vi "Main.vi"(5 "Deliminated Char":string=".", 6 "IGN Folder names":string[](array[string])=["StaARx#[PLC]StaATesterRxSignals", "StaATx#[PLC]StaATesterTxSignals"], 7 "IGN FGVname":string="OPC Ref", 8 "error in":errorcluster, 9 "Sequence Context In":refnum<k7>, 10 "Event Sources":T3, 11 "Ignition In":refnum<class "Ignition.lvclass">) -> (0 "error out":errorcluster, 2 "Station":string="asdfasdf", 3 "Ignition Out":refnum<class "Ignition.lvclass">)   [LabVIEW 2021, in "OPC UA.lvlib" / "Ignition.lvclass"]
uses:
  Ignition.lvclass
  Ignition.lvclass/Ignition.ctl
  OPC UA/OPC UA.lvclass
  Controls/Tester Rx.ctl
  Controls/Tester Tx.ctl
  <vilib>/addons/TestStand/_TSUtility.llb/TestStand - Get Property Value (Number {Signed 32-bit Integer}).vi
panel:
  out "Connect?":bool
  out "Tester Rx":T1
  in  "Tester Tx":T2
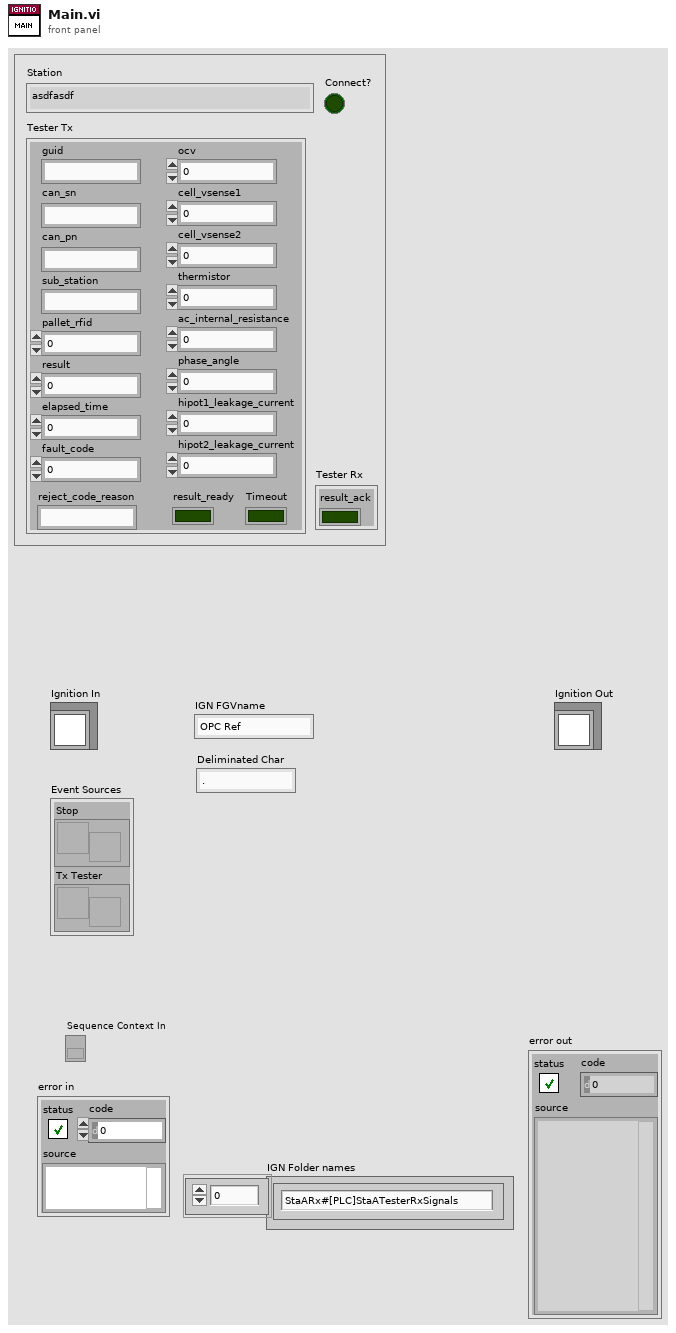
[diagram p1: front panel]
types:
  T1 = typedef "OPC UA.lvlib/Ignition.lvclass/Tester Rx.ctl" = cluster{"result_ack":bool}
  T2 = typedef "OPC UA.lvlib/Ignition.lvclass/Tester Tx.ctl" = cluster{"thermistor":dbl, "phase_angle":dbl, "pallet_rfid":dbl, "ocv":dbl, "cell_vsense1":dbl, "cell_vsense2":dbl, "hipot1_leakage_current":dbl, "hipot2_leakage_current":dbl, "guid":string, "can_sn":string, "can_pn":string, "ac_internal_resistance":dbl, "sub_station":string, "fault_code":i32, "elapsed_time":i32, "result":i32, "reject_code_reason":string, "result_ready":bool, "Timeout":bool}
  T3 = cluster{"Stop":refnum<user-event>, "Tx Tester":refnum<user-event>}
  T4 = cluster{"Stop":refnum<user-event>, "Variant":refnum<user-event>}
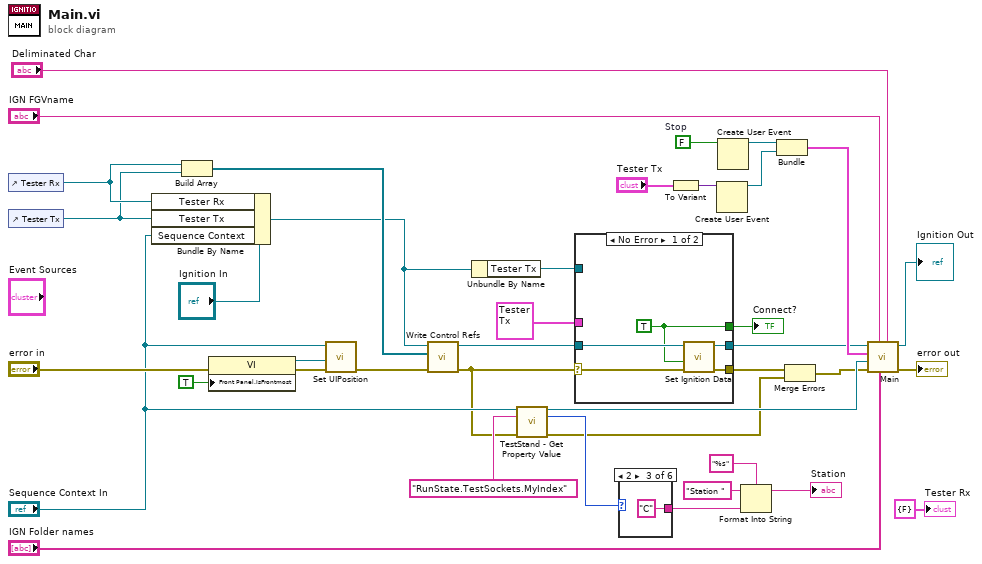
[diagram p0: block diagram]
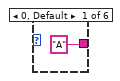
[diagram p2: hidden frame]
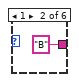
[diagram p3: hidden frame]
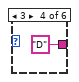
[diagram p4: hidden frame]
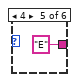
[diagram p5: hidden frame]
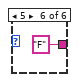
[diagram p6: hidden frame]
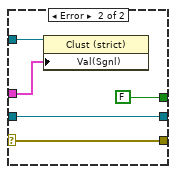
[diagram p7: hidden frame]
diagram:
  w23 = FALSE  # Stop
  n1 = control-ref of="Tester Rx"() -> (w34:refnum<vi>)
  n2 = control-ref of="Tester Tx"() -> (w33:refnum<vi>)
  n3 = Bundle By Name(cluster="Ignition In", "Tester Rx"=w34, "Tester Tx"=w33, "Sequence Context"="Sequence Context In") -> (w15:refnum<class "Ignition.lvclass">)
  n4 = Build Array(w34, w33) -> (w32:refnum<vi>[])
  n5 = property class="VI"(error in="error in", "Front Panel.IsFrontmost"=TRUE ("Front Panel Window:Is Frontmost")) -> (reference out=w27:refnum<vi>, error out=w28:errorcluster)  [unwired: 1 in]
  n6 = call "Set UIPosition.vi"("error in"=w28, "VI Ref"=w27, "Sequence Context In"="Sequence Context In") -> ("error out"=w30:errorcluster)  [unwired: 8 in]
  n7 = call-dynamic "Write Control Refs.vi"("error in (no error)"=w30, "Ctl Refs"=w32, "OPC UA in"=w15) -> ("error out"=w4:errorcluster, "OPC UA out"=w25:refnum<class "Ignition.lvclass">)  [unwired: 7 in]
  n8 = Unbundle By Name(w15) -> ("Tester Tx"=w14:refnum<vi>)
  n9 = call-poly <vilib>:"TestStand - Get Property Value.vi"("Sequence Context In"="Sequence Context In", "Lookup String"="RunState.TestSockets.MyIndex", "error in (no error)"=w4) -> ("Sequence Context Out"=w5:refnum<k7>, "Value"=w8:i32, "error out"=w2:errorcluster)  [unwired: 10 in]
  n10 = case shown="No Error" w4 {
    selector: w4 -> [w41 w47]
    tunnel: [w44 w47] -> w26
    tunnel: w25 -> [w43 w48]
    tunnel: [w42 w48] -> w18
    tunnel: [w40 FALSE ("result_ready")] -> w16
    tunnel: w14 -> [_ w46]
    tunnel: T2 {"thermistor"=0.0, "phase_angle"=0.0, "pallet_rfid"=0.0, "ocv"=0.0, "cell_vsense1"=0.0, "cell_vsense2"=0.0, "hipot1_leakage_current"=0.0, "hipot2_leakage_current"=0.0, "guid"="", "can_sn"="", "can_pn"="", "ac_internal_resistance"=0.0, "sub_station"="", "fault_code"=0, "elapsed_time"=0, "result"=0, "reject_code_reason"="", "result_ready"=FALSE, "Timeout"=FALSE} ("Value (Signaling)") -> [_ w45]
    frame No Error {
      w40 = TRUE ("result_ready")
      n11 = call "Set Ignition Data.vi"("error in"=w41, "result_ready"=w40, "Ignition in"=w43) -> ("error out"=w44:errorcluster, "Ignition out"=w42:refnum<class "Ignition.lvclass">)  [unwired: 7 in]
    }
    frame Error {
      n12 = property class="Clust (strict)"(reference=w46, "Val(Sgnl)"=w45) -> ()  [unwired: 1 in, 2 out]
    }
  }
  "Connect?" <- w16
  n13 = case shown="2" w8 {
    tunnel: ["A" ("format string") "B" ("format string") "C" ("format string") "D" ("format string") "E" ("format string") "F" ("format string")] -> w7
    frame 0, Default {
    }
    frame 1 {
    }
    frame 2 {
    }
    frame 3 {
    }
    frame 4 {
    }
    frame 5 {
    }
  }
  n14 = To Variant(anything="Tester Tx") -> (Variant=w21:variant)
  n15 = Create User Event(user event datatype=w21) -> (user event=w24:refnum<user-event>)  [unwired: 1 in, 1 out]
  n16 = Create User Event(user event datatype=w23) -> (user event=w22:refnum<user-event>)  [unwired: 1 in, 1 out]
  n17 = Format Into String(format string="%s", initial string="Station ", w7) -> (resulting string=→"Station":string)  [unwired: 1 in, 1 out]
  n18 = Bundle("Stop"=w22, "Variant"=w24) -> (w19:T4)  [unwired: 1 in]
  n19 = Merge Errors(w26, w2) -> (w3:errorcluster)
  n20 = call-parent "Main.vi"("Deliminated Char"="Deliminated Char", "Folder names"="IGN Folder names", "FGVname"="IGN FGVname", "error in"=w3, "Sequence Context In"=w5, "Event Sources"=w19, "OPC UA In"=w18) -> ("error out"=→"error out":errorcluster, "OPC UA Out"=→"Ignition Out":refnum<class "Ignition.lvclass">)  [unwired: 2 in, 1 out]
  "Tester Rx" <- T1 {"result_ack"=FALSE} ("Tester Rx")
